vi "Convert CAN Arb ID to J1939 ID.vi"(0 "Arb ID":u32 format="%.0x") -> (4 "Priority":u8=6, 8 "PGN Fields":T1={"Reserved Bit"=0, "Data page"=0, "PDU Format"=254, "PDU Specific"=250}, 10 "PGN":u32 format="%.0x", 15 "Source Address":u8=27)   [LabVIEW 2023, in "J1939 Utilities.lvlib"]
uses:
  J1939 Utilities.lvlib
  Types/PGN Fields Cluster.ctl
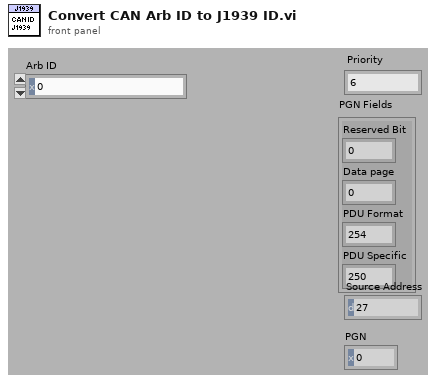
[diagram p1: front panel]
types:
  T1 = typedef "J1939 Utilities.lvlib/PGN Fields Cluster.ctl" = cluster{"Reserved Bit":u8, "Data page":u8, "PDU Format":u8, "PDU Specific":u8}
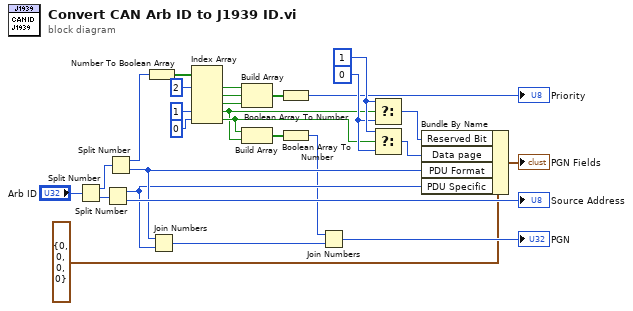
[diagram p0: block diagram]
diagram:
  w18 = u8 0 ("x")
  w19 = u8 1 ("x")
  n1 = Split Number(x="Arb ID") -> (hi(x)=w26:u16, lo(x)=w27:u16)
  n2 = Split Number(x=w27) -> (hi(x)=w23:u8, lo(x)=→"Source Address":u8)
  n3 = Split Number(x=w26) -> (hi(x)=w21:u8, lo(x)=w24:u8)
  n4 = Number To Boolean Array(number=w21) -> (Boolean array=w20:bool[])
  n5 = Join Numbers(hi=w24, lo=w23) -> ((hi.lo)=w9:u16)
  n6 = Index Array(array=w20, index #1=2 ("index"), index #4=1 ("index"), index #5=0 ("index")) -> (element #1=w12:bool, element #2=w13:bool, element #3=w14:bool, element #4=w4:bool, element #5=w5:bool)  [unwired: 2 in]
  n7 = Build Array(w12, w13, w14) -> (w11:bool[])
  n8 = Build Array(w5, w4) -> (w3:bool[])
  n9 = Boolean Array To Number(Boolean array=w11) -> (number=→"Priority":u8)
  n10 = Boolean Array To Number(Boolean array=w3) -> (number=w2:u8)
  n11 = Join Numbers(hi=w2, lo=w9) -> ((hi.lo)=→"PGN":u32)
  n12 = Select(t=w19, s=w4, f=w18) -> (s? t:f=w6:u8)
  n13 = Select(t=w19, s=w5, f=w18) -> (s? t:f=w1:u8)
  n14 = Bundle By Name(cluster=T1 {"Reserved Bit"=0, "Data page"=0, "PDU Format"=0, "PDU Specific"=0} ("PGN Fields"), "Reserved Bit"=w6, "Data page"=w1, "PDU Format"=w24, "PDU Specific"=w23) -> (→"PGN Fields":T1)
